vi "StudentCode.vi"(0 "Sensor 1 Mode":dbl, 1 "Sensor 1 Value":dbl, 2 "Sensor 2 Mode":dbl, 3 "Sensor 2 Value":dbl) -> (15 "Motor 1 Value":dbl, 16 "Motor On Duration":dbl, 18 "Motor 2 Value":dbl)   [LabVIEW 2016]
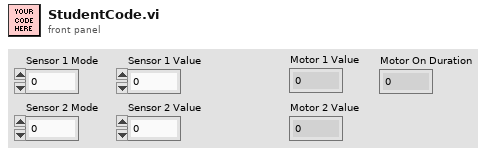
[diagram p1: front panel]
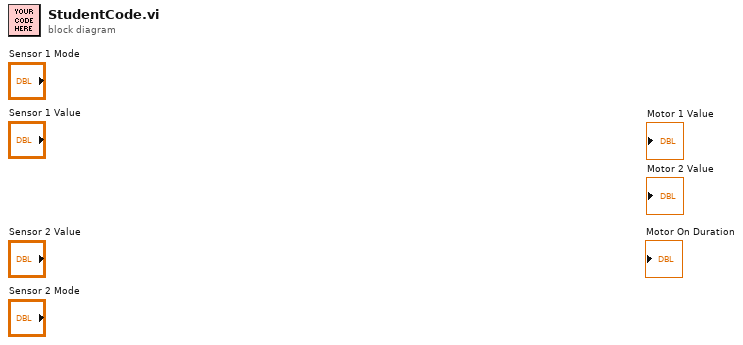
[diagram p0: block diagram]
diagram:
